vi "DB Tools Select Data EDITED.vi"(8 "error_in":errorcluster, 10 "SELECT_statement":string, 11 "connection_reference_in":T1) -> (0 "error_out":errorcluster, 1 "SQL_result":variant[][](array[variant]), 3 "connection_reference_out":T1, 4 "executed_SQL_statement":string)   [LabVIEW 2020]
doc: "This is edited version of DB Tools Select Data vi from NI Database Connectivity Toolkit, with added functionality to limit number of row selected. Also added output with exact SQL statement sent to database. PROCEED WITH CARE (JL)"
uses:
  <vilib>/addons/database/Connection.llb/Conn ObjectReference.ctl
  SQL_statement_type.ctl
  <vilib>/addons/database/Connection.llb/Conn Execute.vi
  <vilib>/addons/database/Recordset.llb/Rec Fetch Recordset Data (R).vi
  <vilib>/addons/database/Recordset.llb/Rec Destroy - Connection.vi
  <vilib>/addons/database/NI_Database_API.lvlib
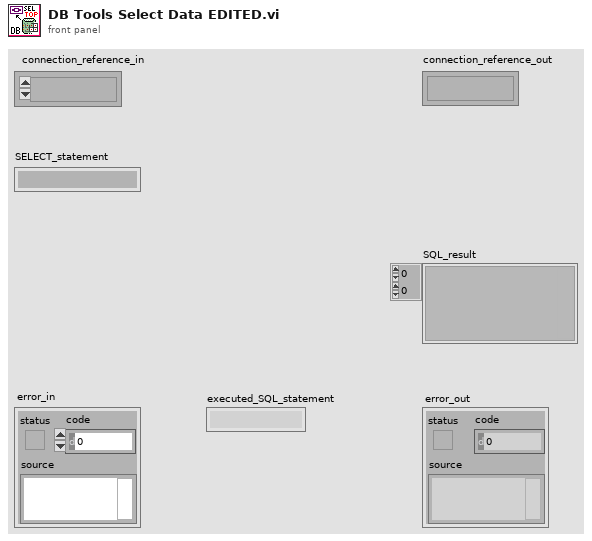
[diagram p1: front panel]
types:
  T1 = typedef "NI_Database_API.lvlib/Conn ObjectReference.ctl" = refnum<k1>
  T2 = typedef "SQL_statement_type.ctl" = enum16{"SELECT", "INSERT", "UPDATE", "DELETE"}
  T3 = typedef "NI_Database_API.lvlib/Rec ObjectReference.ctl" = refnum<k1>
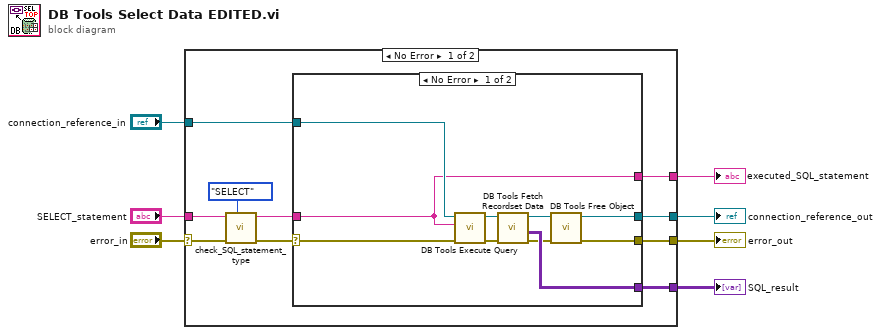
[diagram p0: block diagram]
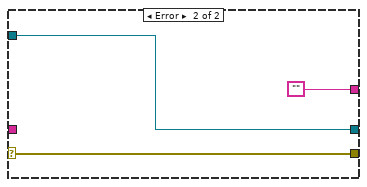
[diagram p2: hidden frame]
diagram:
  n1 = case shown="No Error" "error_in" {
    selector: "error_in" -> [w9 w33]
    tunnel: "SELECT_statement" -> [w12 _]
    tunnel: [w17 w33] -> w6
    tunnel: [w16 _] -> w5
    tunnel: [w15 w32] -> w4
    tunnel: "connection_reference_in" -> [w14 w32]
    tunnel: [w13 ""] -> w1
    frame No Error {
      n2 = call "check_SQL_statement_type.vi"("SQL_statement_type"=SQL_statement_type."SELECT", "error_in"=w9, "SQL_statement_in"=w12) -> ("error_out"=w8:errorcluster, "SQL_statement_out"=w11:string)  [unwired: 7 in]
      n3 = case shown="No Error" w8 {
        selector: w8 -> [w19 w30]
        tunnel: [w20 w30] -> w17
        tunnel: [w27 _] -> w16
        tunnel: [w26 w29] -> w15
        tunnel: w14 -> [w25 w29]
        tunnel: [w18 ""] -> w13
        tunnel: w11 -> [w18 _]
        frame No Error {
          n4 = call-poly <vilib>:"DB Tools Execute Query.vi"("error in (no error)"=w19, "SQL query"=w18, "connection reference"=w25) -> ("error out"=w22:errorcluster, "recordset reference"=w23:T3)  [unwired: 5 in]
          n5 = call-poly <vilib>:"DB Tools Fetch Recordset Data.vi"("error in (no error)"=w22, "recordset reference"=w23) -> ("error out"=w21:errorcluster, "recordset data"=w27:variant[][], "recordset reference out"=w24:T3)  [unwired: 3 in]
          n6 = call-poly <vilib>:"DB Tools Free Object.vi"("error in (no error)"=w21, "recordset reference"=w24) -> ("error out"=w20:errorcluster, "connection reference"=w26:T1)  [unwired: 8 in]
        }
        frame Error {
        }
      }
    }
    frame Error {
    }
  }
  "error_out" <- w6
  "SQL_result" <- w5
  "connection_reference_out" <- w4
  "executed_SQL_statement" <- w1
